vi "From JSON.vi"(8 "error in (no error)":errorcluster, 11 "JSON":string) -> (0 "error out":errorcluster, 1 "<JSON> Elements":string[](array[string]) caption="<JSON>Elements", 2 "Message Type":T1, 3 "JSONMessage":refnum<class "JSONMessage.lvclass">)   [LabVIEW 2020, in "wamplv.lvlib" / "JSONMessage.lvclass"]
uses:
  JSONMessage.lvclass
  TypeDefs/WAMP Message Codes.ctl
  JSONMessage.lvclass/JSONMessage.ctl
  <vilib>/Utility/error.llb/Error Cluster From Error Code.vi
  <vilib>/JDP Science/JSONtext/JSONtext.lvlib
  wamplv.lvlib
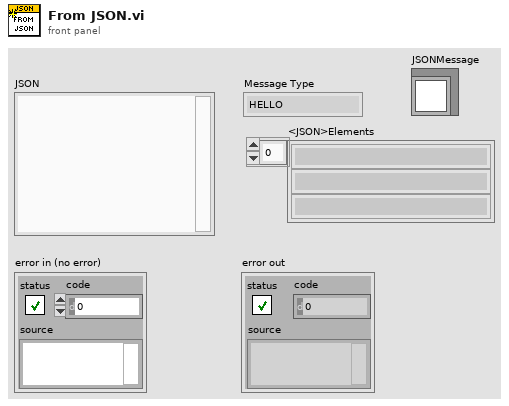
[diagram p1: front panel]
types:
  T1 = typedef "wamplv.lvlib/WAMP Message Codes.ctl" = enum8{"HELLO", "WELCOME", "ABORT", "GOODBYE", "ERROR", "PUBLISH", "PUBLISHED", "SUBSCRIBE", "SUBSCRIBED", "UNSUBSCRIBE", "UNSUBSCRIBED", "EVENT", "CALL", "RESULT", "REGISTER", "REGISTERED", "UNREGISTER", "UNREGISTERED", "INVOCATION", "YIELD"}
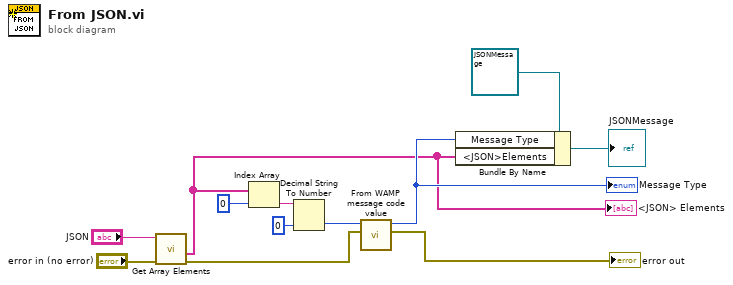
[diagram p0: block diagram]
diagram:
  n1 = call <vilib>:"Get Array Elements.vi"("error in (no error)"="error in (no error)", "JSON"="JSON") -> ("error out"=w4:errorcluster, "<JSON>"=w2:string[])  [unwired: 7 in, 1 out]
  "<JSON> Elements" <- w2
  n2 = Index Array(array=w2, index=0) -> (element=w8:string)
  n3 = Decimal String To Number(string=w8, default (0L)=u8 0 ("default (0 I32)")) -> (number=w6:u8)  [unwired: 1 in, 1 out]
  n4 = call "From WAMP message code value.vi"("error IO"=w4, "WAMP Numeric value"=w6) -> ("error out"=→"error out":errorcluster, "Message Type"=w5:T1)  [unwired: 6 in]
  "Message Type" <- w5
  n5 = Bundle By Name(cluster=refnum<class "JSONMessage.lvclass"> refnum ("wamplv.lvlib:JSONMessage.lvclass"), "Message Type"=w5, "<JSON>Elements"=w2) -> (→"JSONMessage":refnum<class "JSONMessage.lvclass">)
